vi "Master Setup Create Fault Queue.vi"() -> (0 "error out":errorcluster, 3 "Master Fault Queue":refnum<queue>)   [LabVIEW 2017]
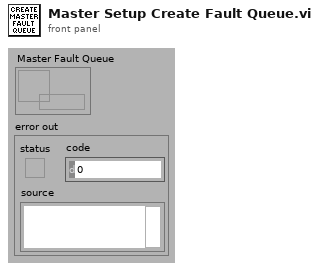
[diagram p1: front panel]
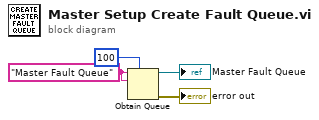
[diagram p0: block diagram]
diagram:
  w2 = "Master Fault Queue" ("name (unnamed)")
  n1 = Obtain Queue(max queue size (-1, unlimited)=100, name (unnamed)=w2, element data type=w2) -> (queue out=→"Master Fault Queue":refnum<queue>, error out=→"error out":errorcluster)  [unwired: 2 in, 1 out]
